vi "SaveData.vi"(0 "Note":string, 1 "GeneralData":bool, 2 "UnitType":T1(ring), 3 "Vin1":dbl, 4 "Vin2":dbl, 5 "Temp1":dbl, 6 "Temp2":dbl, 7 "error in":errorcluster, 8 "CPUTemp":dbl, 9 "refnum in":refnum<file>, 10 "BIT":u32, 12 "time":u32) -> (20 "refnum out":refnum<file>, 27 "error out":errorcluster)   [LabVIEW 2017]
panel:
  out "spreadsheet string":string
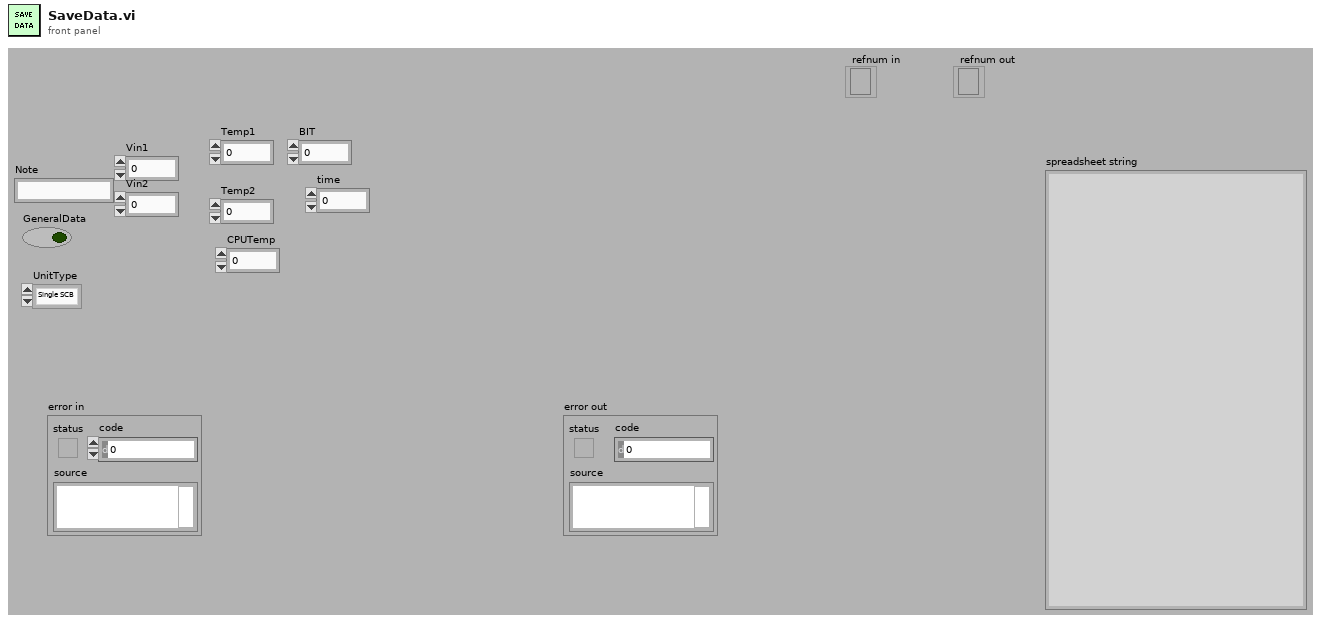
[diagram p1: front panel]
types:
  T1 = enum16{"Single SCB", "Power Rider", "Power Rider&Next10", "HATAL", "DAPH", "Indefinite", "Power Rider 12"}
  T2 = enum16{"open", "replace", "create", "open or create", "replace or create", "replace or create with confirmation"}
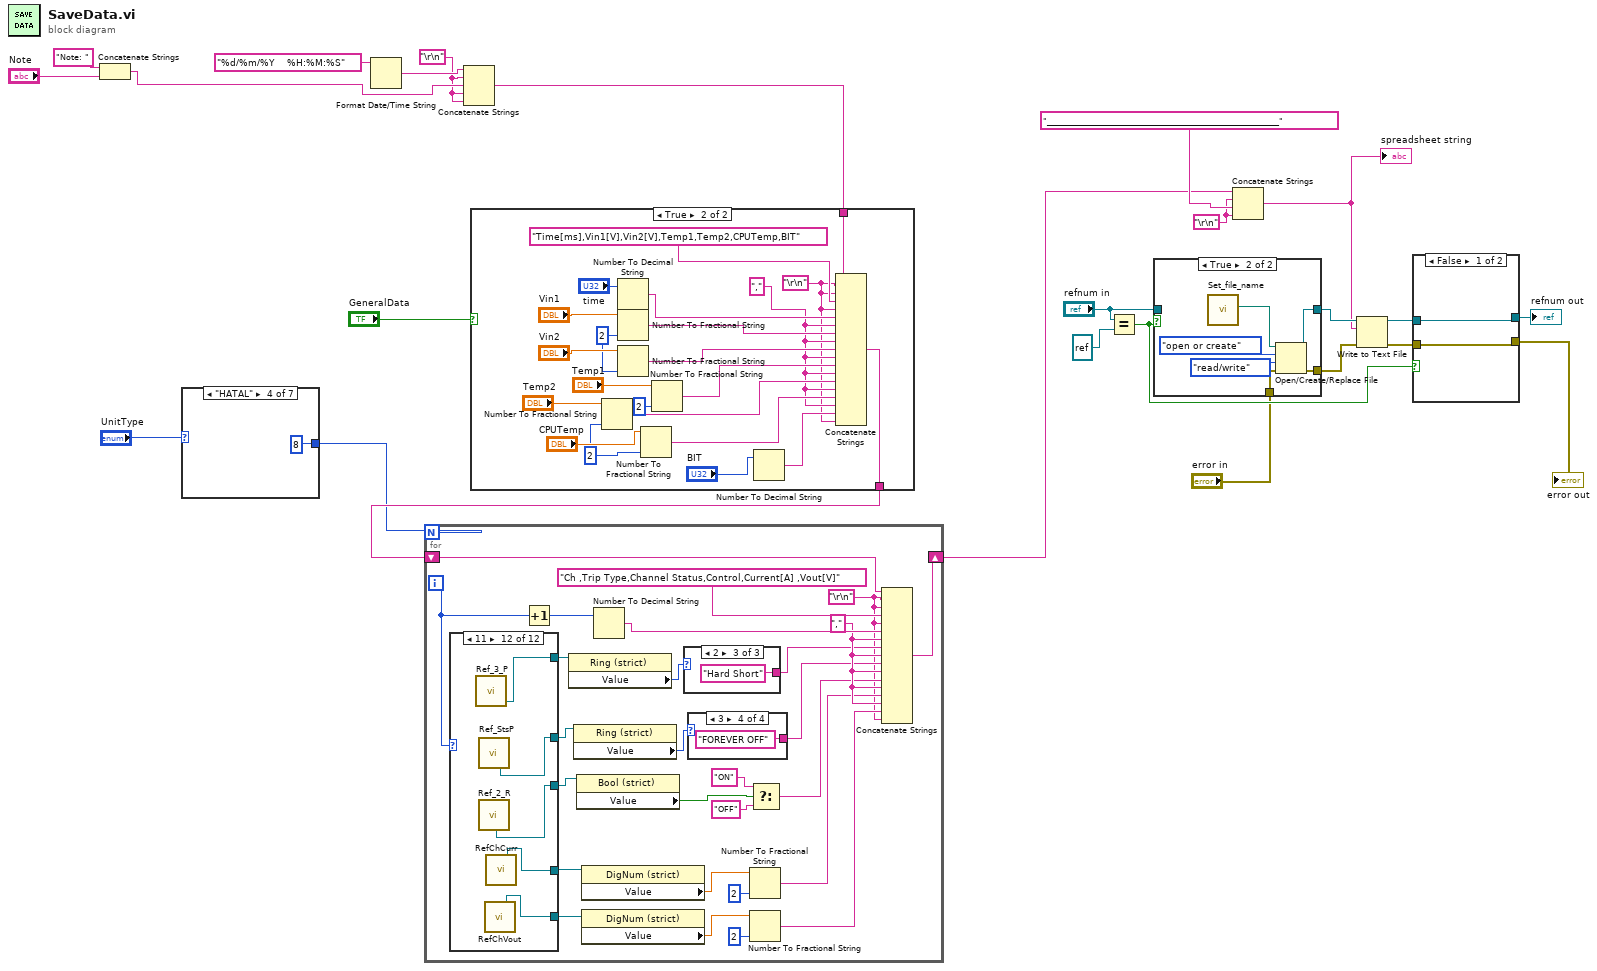
[diagram p0: block diagram]
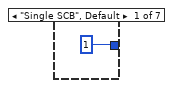
[diagram p2: hidden frame]
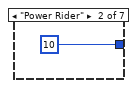
[diagram p3: hidden frame]
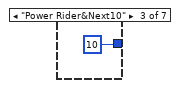
[diagram p4: hidden frame]
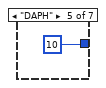
[diagram p5: hidden frame]
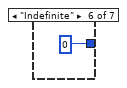
[diagram p6: hidden frame]
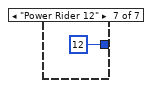
[diagram p7: hidden frame]
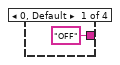
[diagram p8: hidden frame]
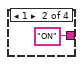
[diagram p9: hidden frame]
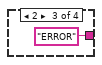
[diagram p10: hidden frame]
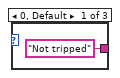
[diagram p11: hidden frame]
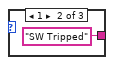
[diagram p12: hidden frame]
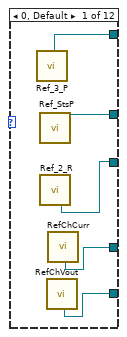
[diagram p13: hidden frame]
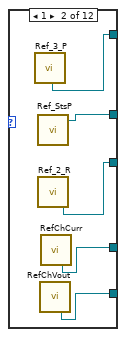
[diagram p14: hidden frame]
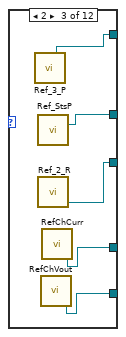
[diagram p15: hidden frame]
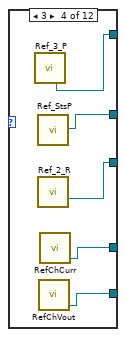
[diagram p16: hidden frame]
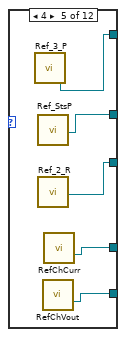
[diagram p17: hidden frame]
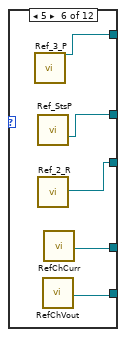
[diagram p18: hidden frame]
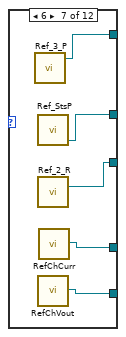
[diagram p19: hidden frame]
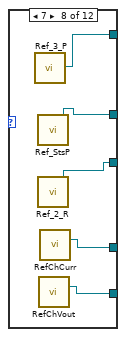
[diagram p20: hidden frame]
diagram:
  w13 = "\r\n"
  w10 = "\r\n"
  n1 = Concatenate Strings("Note: " ("string"), "Note") -> (w21:string)
  n2 = case shown="\"HATAL\"" "UnitType" {
    tunnel: [1 10 10 8 10 0 12] -> w5
    frame "Single SCB", Default {
    }
    frame "Power Rider" {
    }
    frame "Power Rider&Next10" {
    }
    frame "HATAL" {
    }
    frame "DAPH" {
    }
    frame "Indefinite" {
    }
    frame "Power Rider 12" {
    }
  }
  n3 = Format Date/Time String(time format string (%c)="%d/%m/%Y    %H:%M:%S") -> (date/time string=w24:string)  [unwired: 2 in]
  n4 = Concatenate Strings(w24, w10, w21, w10, w10) -> (w11:string)
  n5 = case shown="True" "GeneralData" {
    tunnel: w11 -> [w33 w55]
    tunnel: [w33 w54] -> w8
    frame False {
    }
    frame True {
      w37 = i16 2 ("precision (6)")
      w38 = i16 2 ("precision (6)")
      w39 = ","
      w34 = "\r\n"
      n6 = Number To Fractional String(number="Temp2", precision (6)=w37) -> (F-format string=w44:string)  [unwired: 2 in]
      n7 = Number To Decimal String(number="time") -> (decimal integer string=w52:string)  [unwired: 1 in]
      n8 = Number To Fractional String(number="Vin1", precision (6)=w38) -> (F-format string=w50:string)  [unwired: 2 in]
      n9 = Number To Fractional String(number="Vin2", precision (6)=w38) -> (F-format string=w48:string)  [unwired: 2 in]
      n10 = Number To Fractional String(number="CPUTemp", precision (6)=w37) -> (F-format string=w42:string)  [unwired: 2 in]
      n11 = Number To Fractional String(number="Temp1", precision (6)=i16 2) -> (F-format string=w47:string)  [unwired: 2 in]
      n12 = Number To Decimal String(number="BIT") -> (decimal integer string=w40:string)  [unwired: 1 in]
      n13 = Concatenate Strings(w55, w34, w34, "Time[ms],Vin1[V],Vin2[V],Temp1,Temp2,CPUTemp,BIT" ("string"), w34, w52, w39, w50, w39, w48, w39, w47, w39, w44, w39, w42, w39, w40, w34) -> (w54:string)
    }
  }
  n14 = for {
    N: w5 -> [_]
    shift-right: [w80] -> w7
    shift-left: w8 -> [w81]
    i -> [w76]
    w77 = ","
    w56 = "\r\n"
    n15 = case shown="11" w76 {
      tunnel: [w94 w99 w104 w107 w114 w119 w124 w129 w134 w139 w144 w149] -> w75
      tunnel: [w93 w98 w103 w108 w113 w118 w123 w128 w133 w138 w143 w148] -> w72
      tunnel: [w92 w97 w102 w109 w112 w117 w122 w127 w132 w137 w142 w147] -> w69
      tunnel: [w91 w96 w101 w106 w111 w116 w121 w126 w131 w136 w141 w146] -> w64
      tunnel: [w90 w95 w100 w105 w110 w115 w120 w125 w130 w135 w140 w145] -> w63
      frame 0, Default {
        n16 = call "Ref_3_P.vi"() -> ("Trip  Ch 1 out"=w94:refnum<vi>)  [unwired: 16 in, 11 out]
        n17 = call "Ref_StsP.vi"() -> ("Status Ch1 out"=w93:refnum<vi>)  [unwired: 16 in, 11 out]
        n18 = call "Ref_2_R.vi"() -> ("Control  Ch 1 out"=w92:refnum<vi>)  [unwired: 15 in, 12 out]
        n19 = call "RefChVout.vi"() -> ("Vout  P1 out"=w90:refnum<vi>)  [unwired: 15 in, 12 out]
        n20 = call "RefChCurr.vi"() -> ("Current P1 out"=w91:refnum<vi>)  [unwired: 15 in, 12 out]
      }
      frame 1 {
        n21 = call "Ref_3_P.vi"() -> ("Trip  Ch 2 out"=w99:refnum<vi>)  [unwired: 16 in, 11 out]
        n22 = call "Ref_StsP.vi"() -> ("Status Ch2 out"=w98:refnum<vi>)  [unwired: 16 in, 11 out]
        n23 = call "Ref_2_R.vi"() -> ("Control  Ch 2 out"=w97:refnum<vi>)  [unwired: 15 in, 12 out]
        n24 = call "RefChVout.vi"() -> ("Vout  P2 out"=w95:refnum<vi>)  [unwired: 15 in, 12 out]
        n25 = call "RefChCurr.vi"() -> ("Current P2 out"=w96:refnum<vi>)  [unwired: 15 in, 12 out]
      }
      frame 2 {
        n26 = call "Ref_3_P.vi"() -> ("Trip  Ch 3 out"=w104:refnum<vi>)  [unwired: 16 in, 11 out]
        n27 = call "Ref_StsP.vi"() -> ("Status Ch3 out"=w103:refnum<vi>)  [unwired: 16 in, 11 out]
        n28 = call "Ref_2_R.vi"() -> ("Control  Ch 3 out"=w102:refnum<vi>)  [unwired: 15 in, 12 out]
        n29 = call "RefChVout.vi"() -> ("Vout  P3 out"=w100:refnum<vi>)  [unwired: 15 in, 12 out]
        n30 = call "RefChCurr.vi"() -> ("Current P3 out"=w101:refnum<vi>)  [unwired: 15 in, 12 out]
      }
      frame 3 {
        n31 = call "Ref_3_P.vi"() -> ("Trip  Ch 4 out"=w107:refnum<vi>)  [unwired: 16 in, 11 out]
        n32 = call "Ref_StsP.vi"() -> ("Status Ch4 out"=w108:refnum<vi>)  [unwired: 16 in, 11 out]
        n33 = call "Ref_2_R.vi"() -> ("Control  Ch 4 out"=w109:refnum<vi>)  [unwired: 15 in, 12 out]
        n34 = call "RefChVout.vi"() -> ("Vout  P4 out"=w105:refnum<vi>)  [unwired: 15 in, 12 out]
        n35 = call "RefChCurr.vi"() -> ("Current P4 out"=w106:refnum<vi>)  [unwired: 15 in, 12 out]
      }
      frame 4 {
        n36 = call "Ref_3_P.vi"() -> ("Trip  Ch 5 out"=w114:refnum<vi>)  [unwired: 16 in, 11 out]
        n37 = call "Ref_StsP.vi"() -> ("Status Ch5 out"=w113:refnum<vi>)  [unwired: 16 in, 11 out]
        n38 = call "Ref_2_R.vi"() -> ("Control  Ch 5 out"=w112:refnum<vi>)  [unwired: 15 in, 12 out]
        n39 = call "RefChVout.vi"() -> ("Vout  P5 out"=w110:refnum<vi>)  [unwired: 15 in, 12 out]
        n40 = call "RefChCurr.vi"() -> ("Current P5 out"=w111:refnum<vi>)  [unwired: 15 in, 12 out]
      }
      frame 5 {
        n41 = call "Ref_3_P.vi"() -> ("Trip  Ch 6 out"=w119:refnum<vi>)  [unwired: 16 in, 11 out]
        n42 = call "Ref_StsP.vi"() -> ("Status Ch6 out"=w118:refnum<vi>)  [unwired: 16 in, 11 out]
        n43 = call "Ref_2_R.vi"() -> ("Control  Ch 6 out"=w117:refnum<vi>)  [unwired: 15 in, 12 out]
        n44 = call "RefChVout.vi"() -> ("Vout  P6 out"=w115:refnum<vi>)  [unwired: 15 in, 12 out]
        n45 = call "RefChCurr.vi"() -> ("Current P6 out"=w116:refnum<vi>)  [unwired: 15 in, 12 out]
      }
      frame 6 {
        n46 = call "Ref_3_P.vi"() -> ("Trip  Ch 7 out"=w124:refnum<vi>)  [unwired: 16 in, 11 out]
        n47 = call "Ref_StsP.vi"() -> ("Status Ch7 out"=w123:refnum<vi>)  [unwired: 16 in, 11 out]
        n48 = call "Ref_2_R.vi"() -> ("Control  Ch 7 out"=w122:refnum<vi>)  [unwired: 15 in, 12 out]
        n49 = call "RefChVout.vi"() -> ("Vout  P7 out"=w120:refnum<vi>)  [unwired: 15 in, 12 out]
        n50 = call "RefChCurr.vi"() -> ("Current P7 out"=w121:refnum<vi>)  [unwired: 15 in, 12 out]
      }
      frame 7 {
        n51 = call "Ref_3_P.vi"() -> ("Trip  Ch 8 out"=w129:refnum<vi>)  [unwired: 16 in, 11 out]
        n52 = call "Ref_StsP.vi"() -> ("Status Ch9 out"=w128:refnum<vi>)  [unwired: 16 in, 11 out]
        n53 = call "Ref_2_R.vi"() -> ("Control  Ch 9 out"=w127:refnum<vi>)  [unwired: 15 in, 12 out]
        n54 = call "RefChVout.vi"() -> ("Vout  P8 out"=w125:refnum<vi>)  [unwired: 15 in, 12 out]
        n55 = call "RefChCurr.vi"() -> ("Current P8 out"=w126:refnum<vi>)  [unwired: 15 in, 12 out]
      }
      frame 8 {
        n56 = call "Ref_3_P.vi"() -> ("Trip  Ch 9 out"=w134:refnum<vi>)  [unwired: 16 in, 11 out]
        n57 = call "Ref_StsP.vi"() -> ("Status Ch9 out"=w133:refnum<vi>)  [unwired: 16 in, 11 out]
        n58 = call "Ref_2_R.vi"() -> ("Control  Ch 9 out"=w132:refnum<vi>)  [unwired: 15 in, 12 out]
        n59 = call "RefChVout.vi"() -> ("Vout  P9 out"=w130:refnum<vi>)  [unwired: 15 in, 12 out]
        n60 = call "RefChCurr.vi"() -> ("Current P9 out"=w131:refnum<vi>)  [unwired: 15 in, 12 out]
      }
      frame 9 {
        n61 = call "Ref_3_P.vi"() -> ("Trip  Ch 10 out"=w139:refnum<vi>)  [unwired: 16 in, 11 out]
        n62 = call "Ref_StsP.vi"() -> ("Status Ch10 out"=w138:refnum<vi>)  [unwired: 16 in, 11 out]
        n63 = call "Ref_2_R.vi"() -> ("Control  Ch 10 out"=w137:refnum<vi>)  [unwired: 15 in, 12 out]
        n64 = call "RefChVout.vi"() -> ("Vout  P10 out"=w135:refnum<vi>)  [unwired: 15 in, 12 out]
        n65 = call "RefChCurr.vi"() -> ("Current P10 out"=w136:refnum<vi>)  [unwired: 15 in, 12 out]
      }
      frame 10 {
        n66 = call "Ref_3_P.vi"() -> ("Trip  Ch 11 out"=w144:refnum<vi>)  [unwired: 16 in, 11 out]
        n67 = call "Ref_StsP.vi"() -> ("Status Ch11 out"=w143:refnum<vi>)  [unwired: 16 in, 11 out]
        n68 = call "Ref_2_R.vi"() -> ("Control  Ch 11 out"=w142:refnum<vi>)  [unwired: 15 in, 12 out]
        n69 = call "RefChVout.vi"() -> ("Vout  P11 out"=w140:refnum<vi>)  [unwired: 15 in, 12 out]
        n70 = call "RefChCurr.vi"() -> ("Current P11 out"=w141:refnum<vi>)  [unwired: 15 in, 12 out]
      }
      frame 11 {
        n71 = call "Ref_3_P.vi"() -> ("Trip  Ch 12 out"=w149:refnum<vi>)  [unwired: 16 in, 11 out]
        n72 = call "Ref_StsP.vi"() -> ("Status Ch12 out"=w148:refnum<vi>)  [unwired: 16 in, 11 out]
        n73 = call "Ref_2_R.vi"() -> ("Control  Ch 12 out"=w147:refnum<vi>)  [unwired: 15 in, 12 out]
        n74 = call "RefChVout.vi"() -> ("Vout  P12 out"=w145:refnum<vi>)  [unwired: 15 in, 12 out]
        n75 = call "RefChCurr.vi"() -> ("Current P12 out"=w146:refnum<vi>)  [unwired: 15 in, 12 out]
      }
    }
    n76 = Increment(x=w76) -> (x+1=w79:i32)
    n77 = property class="Ring (strict)"(reference=w75) -> ("Value"=w74:u16)  [unwired: 1 in, 2 out]
    n78 = property class="Ring (strict)"(reference=w72) -> ("Value"=w71:u8)  [unwired: 1 in, 2 out]
    n79 = property class="Bool (strict)"(reference=w69) -> ("Value"=w66:bool)  [unwired: 1 in, 2 out]
    n80 = property class="DigNum (strict)"(reference=w64) -> ("Value"=w62:dbl)  [unwired: 1 in, 2 out]
    n81 = property class="DigNum (strict)"(reference=w63) -> ("Value"=w60:dbl)  [unwired: 1 in, 2 out]
    n82 = Number To Decimal String(number=w79) -> (decimal integer string=w78:string)  [unwired: 1 in]
    n83 = case shown="2" w74 {
      tunnel: ["Not tripped" ("string") "SW Tripped" ("string") "Hard Short" ("string")] -> w73
      frame 0, Default {
      }
      frame 1 {
      }
      frame 2 {
      }
    }
    n84 = case shown="3" w71 {
      tunnel: ["OFF" ("string") "ON" ("string") "ERROR" ("string") "FOREVER OFF" ("string")] -> w70
      frame 0, Default {
      }
      frame 1 {
      }
      frame 2 {
      }
      frame 3 {
      }
    }
    n85 = Number To Fractional String(number=w62, precision (6)=i16 2) -> (F-format string=w61:string)  [unwired: 2 in]
    n86 = Number To Fractional String(number=w60, precision (6)=i16 2) -> (F-format string=w59:string)  [unwired: 2 in]
    n87 = Select(t="ON" ("string"), s=w66, f="OFF" ("string")) -> (s? t:f=w65:string)
    n88 = Concatenate Strings(w81, w56, w56, "Ch ,Trip Type,Channel Status,Control,Current[A] ,Vout[V]" ("string"), w56, w78, w77, w73, w77, w70, w77, w65, w77, w61, w77, w59, w56) -> (w80:string)
  }
  n89 = Equal?(x="refnum in", y=refnum<file> refnum ("refnum out 2")) -> (x = y?=w15:bool)
  n90 = case shown="True" w15 {
    tunnel: "refnum in" -> [w151 _]
    tunnel: [w151 w155] -> w18
    tunnel: "error in" -> [w150 w153]
    tunnel: [w150 w152] -> w3
    frame False {
    }
    frame True {
      n91 = call "Set_file_name.vi"() -> ("appended path"=w154:path)  [unwired: 11 in]
      n92 = Open/Create/Replace File(file path (use dialog)=w154, error in=w153, operation (0:open)=T2."open or create", access (0:read/write)=enum16{"read/write", "read-only", "write-only"}."read/write") -> (refnum out=w155:refnum<file>, error out=w152:errorcluster)  [unwired: 2 in, 1 out]
    }
  }
  n93 = Concatenate Strings(w7, w13, "__________________________________________________________", w13) -> (w12:string)
  "spreadsheet string" <- w12
  n94 = Write to Text File(file (use dialog)=w18, text=w12, error in=w3) -> (refnum out=w17:refnum<file>, error out=w2:errorcluster)  [unwired: 1 in, 1 out]
  n95 = case shown="False" w15 {
    tunnel: w17 -> [w159 w163]
    tunnel: [w159 refnum<file> refnum ("refnum out")] -> w16
    tunnel: w2 -> [w158 w161]
    tunnel: [w158 w160] -> w1
    frame False {
    }
    frame True {
      n96 = Close File(refnum=w163, error in=w161) -> (error out=w160:errorcluster)  [unwired: 1 out]
    }
  }
  "refnum out" <- w16
  "error out" <- w1
